vi "ep_Power Correction (IEEE).vi"(7 "coefficients for correction":cluster{"P1":dbl, "P2":dbl}, 8 "error in (no error)":errorcluster, 9 "voltage MN values":dbl[](array[numeric]), 10 "voltage RMS values":dbl[](array[numeric]), 11 "power values":T1[](array[typedef])) -> (0 "error out":errorcluster, 2 "corrected active power":dbl[](array[numeric]), 3 "dup power values":T1[](array[typedef]))   [LabVIEW 2024]
doc: "Calibrate the active power according to IEEE C57.12.90-1993."
uses:
  <vilib>/addons/Electrical Power/Basic/Measurement/subVIs/basic_Power Value.ctl
  <vilib>/addons/Electrical Power/Basic/NI_EP_Basic.lvlib
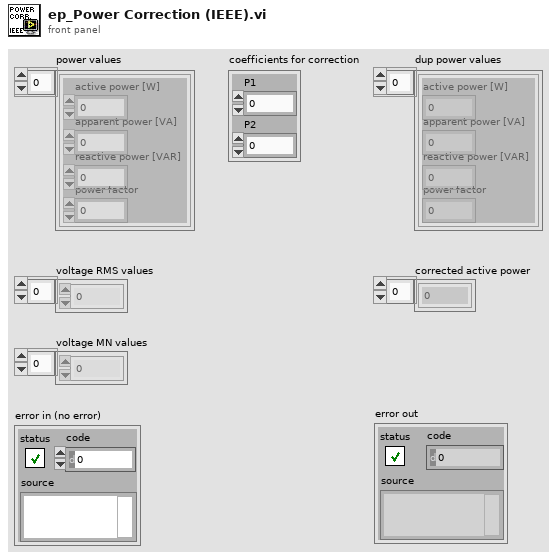
[diagram p1: front panel]
types:
  T1 = typedef "NI_EP_Basic.lvlib/basic_Power Value.ctl" = cluster{"active power [W]":dbl, "apparent power [VA]":dbl, "reactive power [VAR]":dbl, "power factor":dbl}
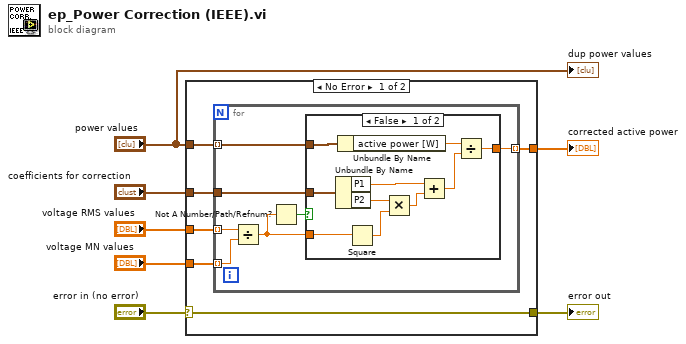
[diagram p0: block diagram]
diagram:
  n1 = case shown="No Error" "error in (no error)" {
    selector: "error in (no error)" -> [w8 w31]
    tunnel: "power values" -> [w13 _]
    tunnel: "coefficients for correction" -> [w12 _]
    tunnel: "voltage RMS values" -> [w11 _]
    tunnel: "voltage MN values" -> [w10 _]
    tunnel: [w9 _] -> w3
    tunnel: [w8 w31] -> w2
    frame No Error {
      n2 = for {
        tunnel: w13 -> [w20] mode=indexing
        tunnel: w12 -> [w19]
        tunnel: w11 -> [w18] mode=indexing
        tunnel: w10 -> [w17] mode=indexing
        tunnel: [w14] -> w9 mode=indexing
        n3 = Divide(x=w18, y=w17) -> (x/y=w16:dbl)
        n4 = Not A Number/Path/Refnum?(number/path/refnum=w16) -> (NaN/Path/Refnum?=w15:bool)
        n5 = case shown="False" w15 {
          tunnel: w20 -> [w30 _]
          tunnel: w19 -> [w29 _]
          tunnel: w16 -> [w28 _]
          tunnel: [w21 _] -> w14
          frame False {
            n6 = Unbundle By Name(w29) -> ("P1"=w25:dbl, "P2"=w27:dbl)
            n7 = Unbundle By Name(w30) -> ("active power [W]"=w23:dbl)
            n8 = Square(x=w28) -> (x^2=w26:dbl)
            n9 = Multiply(x=w27, y=w26) -> (x*y=w24:dbl)
            n10 = Add(x=w25, y=w24) -> (x+y=w22:dbl)
            n11 = Divide(x=w23, y=w22) -> (x/y=w21:dbl)
          }
          frame True {
          }
        }
      }
    }
    frame Error {
    }
  }
  "error out" <- w2
  "corrected active power" <- w3
  "dup power values" <- "power values"
